vi "Agilent Control.vi"() -> ()   [LabVIEW 2014]
uses:
  <instrlib>/Agilent 33XXX Series/Agilent 33XXX Series.lvlib
panel:
  out "VISA resource name out 2":refnum<visa-resource-name>
  out "VISA resource name out":refnum<visa-resource-name>
  in  "VISA resource name 2":refnum<visa-resource-name>
  in  "Duty Cycle (50 %)":i32=50 min=20 max=80
  in  "VISA resource name":refnum<visa-resource-name>
  out "Unit (0: Vpp)":u16(ring) items=["Vpp", "Vrms", "dB"]
  out "error out":errorcluster
  in  "DC Offset (0.00 V)":dbl
  in  "Frequency (1000 Hz)":dbl=1000.0
  in  "Amplitude (1)":dbl=1.0
  in  "Waveform Function (1: Sine)":u16(ring)=1 items=["DC", "Sine", "Square", "Triangle", "Ramp", "Pulse", "Noise", "Sinc", "Negative Ramp", "Exponential Rise", "Exponential Fall", "Cardiac"]
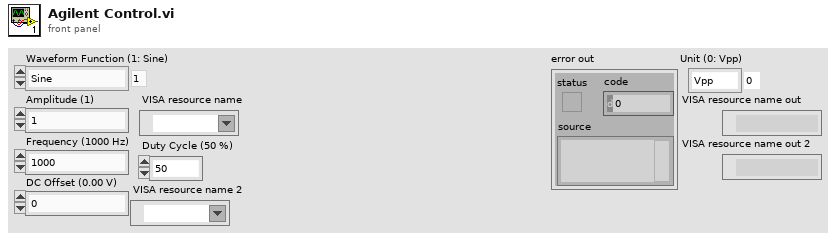
[diagram p1: front panel]
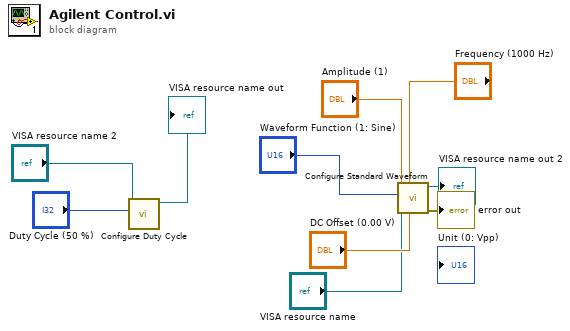
[diagram p0: block diagram]
diagram:
  n1 = call <instrlib>:"Configure Duty Cycle.vi"("Duty Cycle (50 %)"="Duty Cycle (50 %)", "VISA resource name"="VISA resource name 2") -> ("VISA resource name out"=→"VISA resource name out":refnum<visa-resource-name>)  [unwired: 8 in, 1 out]
  n2 = call <instrlib>:"Configure Standard Waveform.vi"("DC Offset (0.00 V)"="DC Offset (0.00 V)", "Frequency (1000 Hz)"="Frequency (1000 Hz)", "Amplitude (1)"="Amplitude (1)", "Waveform Function (1: Sine)"="Waveform Function (1: Sine)", "VISA resource name"="VISA resource name") -> ("error out"=→"error out":errorcluster, "VISA resource name out"=→"VISA resource name out 2":refnum<visa-resource-name>)  [unwired: 5 in]
